vi "ep03_events.vi"() -> ()   [LabVIEW 2019]
panel:
  out "Line String":string
  out "Length":u16
  out "Running":bool
  out "Information":string
  in  "Baud Rate Input":T1(ring)=enum."115200" caption="Baud Rate"
  in  "Port Id Input":T2(ring)=enum."COM3" caption="Port Name"
  in  "stop":bool
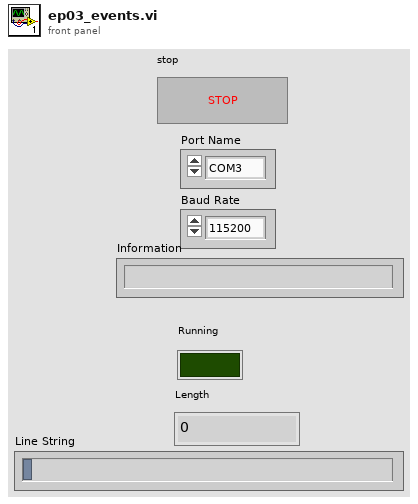
[diagram p1: front panel]
types:
  T1 = enum32{"300", "600", "1200", "2400", "4800", "9600", "14400", "19200", "28800", "38400", "56000", "57600", "115200", "128000", "256000"}
  T2 = enum8{"COM1", "COM2", "COM3", "COM4", "COM5", "COM6", "COM7", "COM8", "COM9", "COM10", "COM11", "COM12", "COM13", "COM14", "COM15", "COM16", "COM17", "COM18", "COM19", "COM20", "COM21", "COM22", "COM23", "COM24", "COM25", "COM26", "COM27", "COM28", "COM29", "COM30", "COM31", "COM32", "COM33", "COM34", "COM35", "COM36", "COM37", "COM38", "COM39", "COM40", "COM41", "COM42", "COM43", "COM44", "COM45", "COM46", "COM47", "COM48"}
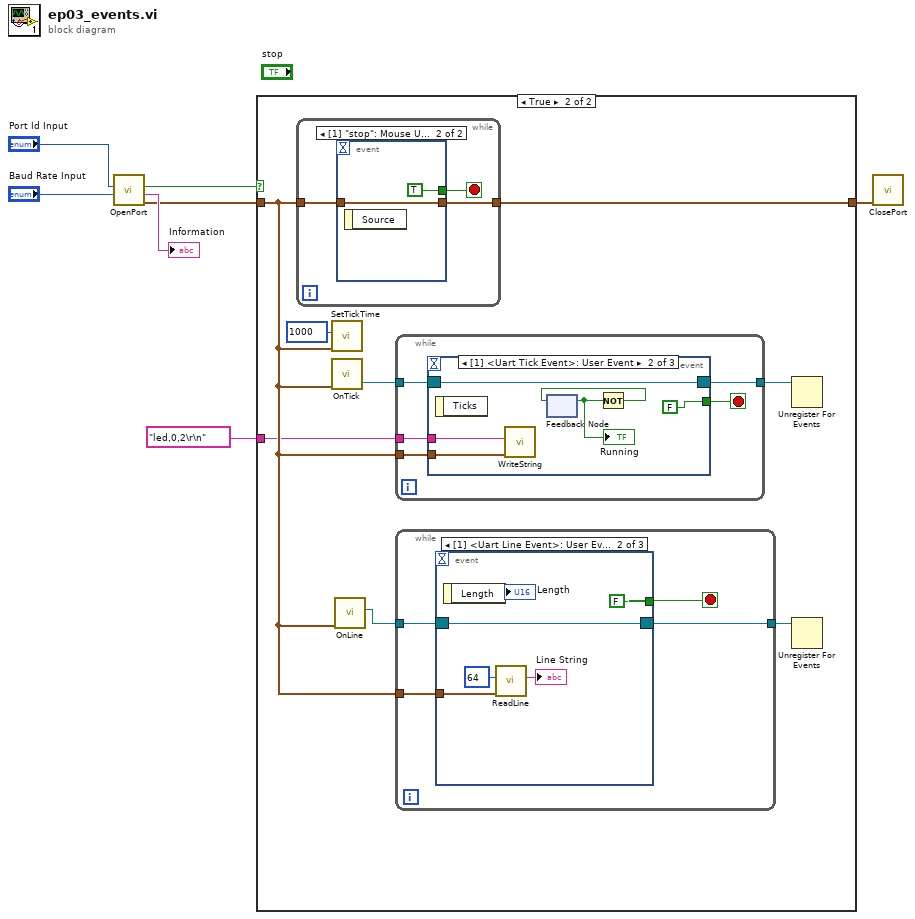
[diagram p0: block diagram]
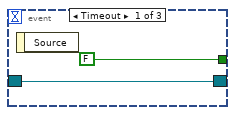
[diagram p3: hidden frame]
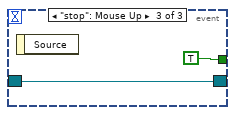
[diagram p4: hidden frame]
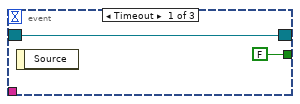
[diagram p5: hidden frame]
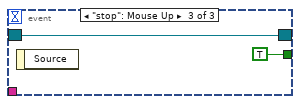
[diagram p6: hidden frame]
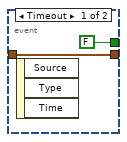
[diagram p7: hidden frame]
diagram:
  n1 = call "OpenPort.vi"("Baud Rate Input"="Baud Rate Input", "Port Id Input"="Port Id Input") -> ("Uart Output"=w3:cluster{u64}, "Information"=→"Information":string, "Port Status"=w5:bool)  [unwired: 6 in, 1 out]
  n2 = case shown="True" w5 {
    tunnel: w3 -> [w8 w10]
    tunnel: [w8 w16] -> w2
    tunnel: "led,0,2\r\n" -> [_ w9]
    frame False {
    }
    frame True {
      n3 = while {
        tunnel: w10 -> [w47]
        tunnel: [w46] -> w16
        stop <- w48 stop-if-true
        n4 = event shown="[1] \"stop\": Mouse Up" {
          selector: _ -> [_ _]
          dyn-events: _ -> [_ _]
          timeout: _ -> [_ _]
          tunnel: [FALSE TRUE] -> w48
          tunnel: w47 -> [w49 w51]
          tunnel: [w49 w51] -> w46
          event Timeout {
            n5 = event-data() -> ()  [unwired: 1 in, 3 out]
          }
          event "stop": Mouse Up {
            n6 = event-data() -> ()  [unwired: 1 in, 1 out]
          }
        }
      }
      n7 = call "SetTickTime.vi"("Uart Input"=w10, "Tick Interval (ms)"=u32 1000) -> ()  [unwired: 8 in, 2 out]
      n8 = call "OnTick.vi"("Uart Input"=w10) -> ("On Tick Event"=w15:refnum<event-registration>)  [unwired: 8 in, 2 out]
      n9 = call "OnLine.vi"("Uart Input"=w10) -> ("On Line Event"=w13:refnum<event-registration>)  [unwired: 8 in, 2 out]
      n10 = while {
        tunnel: w15 -> [w34]
        tunnel: [w33] -> w12
        tunnel: w10 -> [w32]
        tunnel: w9 -> [w31]
        stop <- w35 stop-if-true
        n11 = event shown="[1] <Uart Tick Event>: User Event" {
          selector: w34 -> [w36 w41 w44]
          dyn-events: [w36 w41 w44] -> w33
          timeout: _ -> [_ _ _]
          tunnel: [FALSE FALSE TRUE] -> w35
          tunnel: w32 -> [_ w39 _]
          tunnel: w31 -> [_ w38 _]
          event Timeout {
            n12 = event-data() -> ()  [unwired: 1 in, 1 out]
          }
          event User Event {
            n13 = event-data() -> ()  [unwired: 1 in, 1 out]
            n14 = call "WriteString.vi"("Uart Input"=w39, "String Data"=w38) -> ()  [unwired: 7 in, 3 out]
            n15 = feedback #1() -> (w42:bool)  [unwired: 1 in]
            "Running" <- w42
            n16 = Not(x=w42) -> (.not. x?=w43:bool)
            n17 = feedback-in #1(w43) -> ()
          }
          event "stop": Mouse Up {
            n18 = event-data() -> ()  [unwired: 1 in, 1 out]
          }
        }
      }
      n19 = while {
        tunnel: w13 -> [w19]
        tunnel: [w18] -> w11
        tunnel: w10 -> [w17]
        stop <- w20 stop-if-true
        n20 = event shown="[1] <Uart Line Event>: User Event" {
          selector: w19 -> [w21 w27 w29]
          dyn-events: [w21 w27 w29] -> w18
          timeout: _ -> [_ _ _]
          tunnel: [FALSE FALSE TRUE] -> w20
          tunnel: w17 -> [_ w25 _]
          event Timeout {
            n21 = event-data() -> ()  [unwired: 1 in, 1 out]
          }
          event User Event {
            n22 = event-data() -> ("Length"=→"Length":u16)  [unwired: 1 in]
            n23 = call "ReadLine.vi"("Uart Input"=w25, "Buffer Size (32 bytes)"=u32 64) -> ("Line String"=→"Line String":string)  [unwired: 5 in, 4 out]
          }
          event "stop": Mouse Up {
            n24 = event-data() -> ()  [unwired: 1 in, 1 out]
          }
        }
      }
      n25 = Unregister For Events(event registration refnum=w12) -> ()  [unwired: 1 in, 1 out]
      n26 = Unregister For Events(event registration refnum=w11) -> ()  [unwired: 1 in, 1 out]
    }
  }
  n27 = call "ClosePort.vi"("Uart Input"=w2) -> ()  [unwired: 9 in, 2 out]
